vi "Read Assert Data.vi"(11 "Input in":refnum<class "Input.lvclass">) -> (2 "Assert Data":T1)   [LabVIEW 2016, in "AssertEngine.lvlib" / "Input.lvclass"]
uses:
  Input.lvclass
  Log Assert/Assert Data.ctl
  Input.lvclass/Input.ctl
  AssertEngine.lvlib
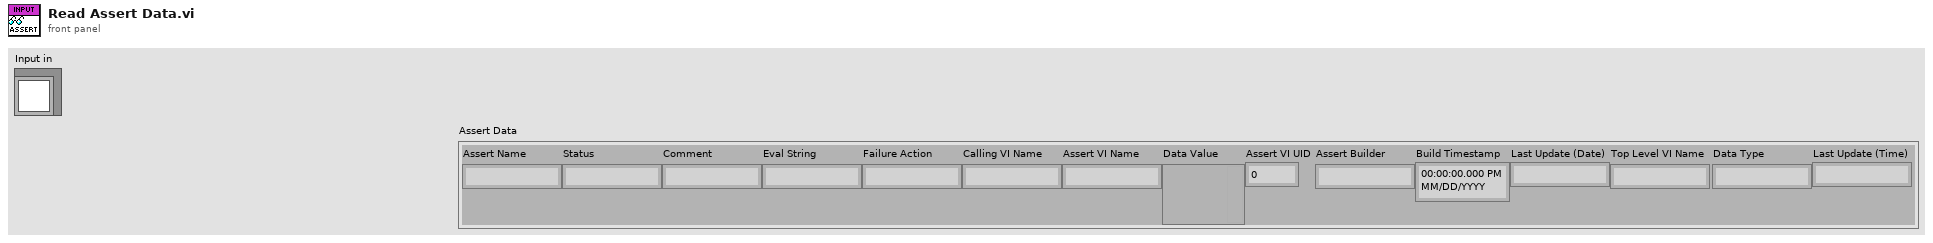
[diagram p1: front panel]
types:
  T1 = typedef "AssertEngine.lvlib/Assert Data.ctl" = cluster{"Assert Name":string, "Status":string, "Comment":string, "Eval String":string, "Failure Action":string, "Calling VI Name":string, "Assert VI Name":string, "Data Value":variant, "Assert VI UID":i32, "Assert Builder":string, "Build Timestamp":timestamp, "Last Update (Date)":string, "Top Level VI Name":string, "Data Type":string, "Last Update (Time)":string}
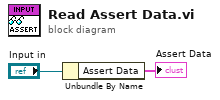
[diagram p0: block diagram]
diagram:
  n1 = Unbundle By Name("Input in") -> ("Assert Data"=→"Assert Data":T1)
